vi "23384_Davis_Poku_Amankwa_Amankwa.DavisPoku.MNE1201.6.DIYa_348261_2031058198.vi"(10 "Integer input":i32) -> (2 "Factorial":ext format="%#_38g")   [LabVIEW 2018]
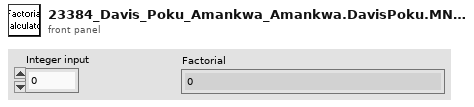
[diagram p1: front panel]
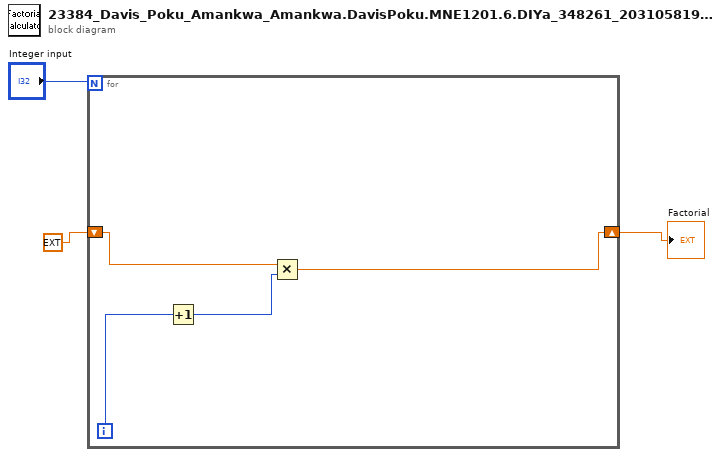
[diagram p0: block diagram]
diagram:
  n1 = for {
    N: "Integer input" -> [_]
    shift-right: [w4] -> w1
    shift-left: ext 1.0 -> [w6]
    i -> [w7]
    n2 = Increment(x=w7) -> (x+1=w5:i32)
    n3 = Multiply(x=w6, y=w5) -> (x*y=w4:ext)
  }
  "Factorial" <- w1
